vi "Caller.vi"(0 "Add in":refnum<class "Add.lvclass">, 2 "DVR":refnum<data-value>, 5 "Sub Panel":refnum<vi>, 7 "Stop":refnum<user-event>, 9 "Class Data":refnum<user-event>, 11 "Error In":errorcluster) -> (4 "Add out":refnum<class "Add.lvclass">, 15 "Error Out":errorcluster)   [LabVIEW 2019, in "Add.lvclass"]
doc: "The VI asynchronously calls the Operation UI method of the addition operation."
uses:
  Add.lvclass
  Operation UI.vi
  Arithemtic Operation/Arithemetic Operation.lvclass
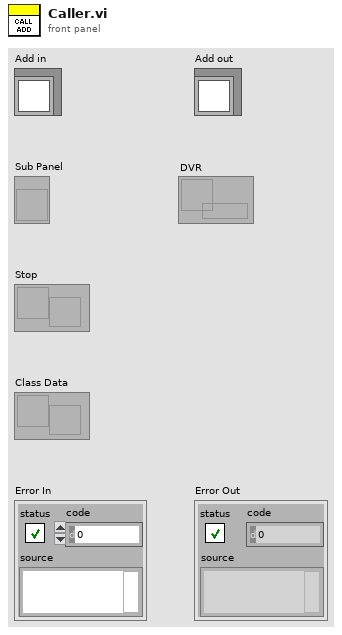
[diagram p1: front panel]
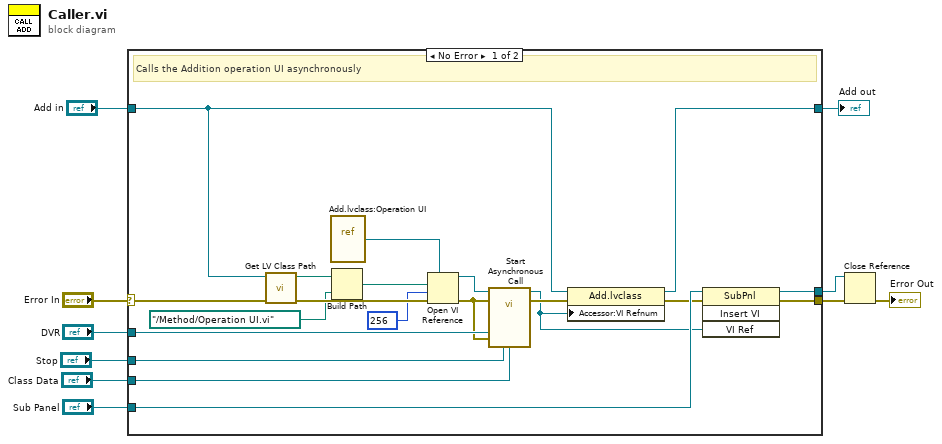
[diagram p0: block diagram]
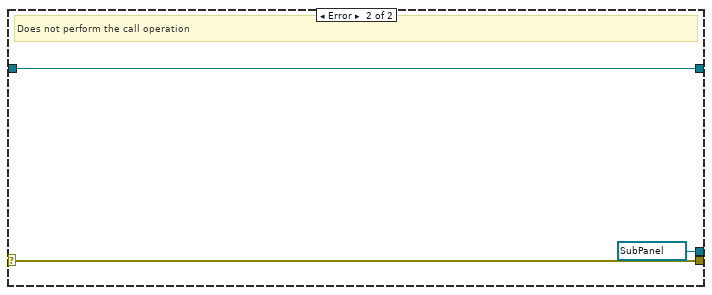
[diagram p2: hidden frame]
diagram:
  n1 = case shown="No Error" "Error In" {
    selector: "Error In" -> [w24 w33]
    tunnel: [w23 w33] -> w9
    tunnel: [w18 w32] -> w7
    tunnel: "Add in" -> [w17 w32]
    tunnel: "Stop" -> [w12 _]
    tunnel: "Class Data" -> [w11 _]
    tunnel: "Sub Panel" -> [w22 _]
    tunnel: [w21 refnum<vi> refnum ("Sub Panel")] -> w2
    tunnel: "DVR" -> [w14 _]
    frame No Error {
      # "Calls the Addition operation UI asynchronously"
      n2 = call <vilib>:"Get LV Class Path.vi"("error in (no error)"=w24, "object"=w17) -> ("error out"=w30:errorcluster, "class path"=w29:path)  [unwired: 8 in]
      n3 = vi-ref "Add.lvclass:Operation UI.vi"() -> (w16:refnum<vi>)
      n4 = Build Path(base path=w29, name or relative path=path "../Method/Operation UI.vi") -> (appended path=w15:path)
      n5 = Open VI Reference(type specifier VI Refnum (for type only)=w16, vi path=w15, options=256, error in (no error)=w30) -> (vi reference=w25:refnum<vi>, error out=w13:errorcluster)  [unwired: 2 in]
      n6 = call-by-ref "Start Asynchronous Call"(reference=w25, error in=w13, "DVR In"=w14, "Error In"=w13, "Stop"=w12, "Class Data"=w11) -> (reference out=w19:refnum<vi>, error out=w27:errorcluster)  [unwired: 9 in, 3 out]
      n7 = property class="Add.lvclass"(reference=w17, error in=w27, "Accessor:VI Refnum"=w19) -> (reference out=w18:refnum<class "Add.lvclass">, error out=w20:errorcluster)
      n8 = invoke class="SubPnl" method="Insert VI"(reference=w22, error in=w20, "VI Ref"=w19) -> (reference out=w21:refnum<vi>, error out=w23:errorcluster)  [unwired: 1 in, 2 out]
    }
    frame Error {
      # "Does not perform the call operation"
    }
  }
  "Add out" <- w7
  n9 = Close Reference(reference=w2, error in (no error)=w9) -> (error out=→"Error Out":errorcluster)
